vi "RVHR - Configure Language.vi"(7 "Directory Path":path, 8 "error in (no error)":errorcluster, 10 "Supervisory Config Cluster Out":T3={"UI Information"={"Header Image"=path "../Data/header.png", "Language"=enum."English", "First Run?"=FALSE, "Setup Camera?"=FALSE, "Device Type"=enum."RCA", "Encoder Type"=enum."Tacho", "Version"=enum."RailMeasurement_CAT", "port"=0, "greyscale"=FALSE, "camera index"=0}, "Test Cluster"={"Operator"="", "Description"="", "Line"="", "Start Position"=450000.0, "Run Length"=31.0, "Sensor A Position"=80000.0, "Rail Side"=FALSE, "Distance Direction"=FALSE, "Path"=path "", "Sensor B Position"=0.0, "Visible Chart Distance"=0.0, "Company"="", "Ref Profile"=""}, "RV-HR Settings Cluster"={"Sensor A Calibration"=0.0, "Integrator Time"=0.0, "Encoder Spacing"=0.0, "Encoder Threshold"=0.0, "Sampling Distance"=0, "Swap Direction?"=FALSE, "Min Walking Speed"=0.0, "Max Walking Speed"=0.0, "Distance Format"=0, "Sensor B Calibration"=0.0, "Tacho Pulses/Rev"=0.0, "Wheel Diameter"=0.0, "Max Short Roughness"=0.0, "Max Long Roughness"=0.0, "Measuring Interval"=0.0, "Measuring Length"=0.0, "Wavelengths"=[], "Device Resolution"=0, "Detect Change in Direction?"=FALSE, "Save Images?"=FALSE, "Image Frequency"=0, "Save Video?"=FALSE, "Image Offset"=0.0, "Start Position at 0m?"=FALSE, "Live Corrug Est.?"=FALSE, "Wavelength Corrug"=0, "Distance Corrug"=0, "Update Corrug"=0}} {"RV-HR Settings Cluster"."Image Frequency" items=["2", "3", "5"]; "RV-HR Settings Cluster"."Device Resolution" items=["0.1 µm", "1 µm", "10 µm"]; "RV-HR Settings Cluster"."Distance Format" items=["kilometres", "miles & chains", "metres", "stations", "miles"]; "RV-HR Settings Cluster"."Sampling Distance" items=["1mm", "2mm"]}, 11 "UI References":T13) -> (0 "error out":errorcluster, 1 "UI Information.Language":T1, 2 "Language Config Cluster Out":T2={"Home"="Home", "Test Setup"="Setup", "Run Test"="Test", "Configure"="Config", "Hardware Viewer"="Viewer", "Review Test"="Review", "Report"="Home", "Exit"="Exit", "Device Connected?"="Device Connected?", "Test in Progress?"="Test in Progress?", "Simulate?"="Simulate?", "Device Type 1"="Corrugation Analysis Trolley", "Device Type 2"="Bi-Corrugation Analysis Trolley", "Device Type 3"="Bi-Corrugation Analysis Trolley", "Device Type 4"="Bi-Corrugation Analysis Trolley", "Device Type 5"="Bi-Corrugation Analysis Trolley", "Device Type 6"="Bi-Corrugation Analysis Trolley", "Device Type 7"="Bi-Corrugation Analysis Trolley", "Software Version"="Version", "Support"="Software by RailMeasurement Limited - Cambridge - UK - support@railmeasurement.com", "Operator"="Operator:", "Test Description"="Description:", "Line"="Description:", "Test Folder Path"="Folder Path:", "Test Folder Path RCA"="Folder Path:", "Start Position"="Start Position:", "Sensor Position"="Sensor Position:", "Sensor A Position"="Sensor A Position:", "Sensor B Position"="Sensor B Position:", "Visible Chart Distance"="Sensor B Position:", "Rail Side"="Rail Side:", "Rail A Side"="Rail A Side:", "Distance Direction"="Distance Direction:", "Start"="Start:", "Distance Travelled"="Distance Travelled:", "Current Position"="Current Position:", "Stop Test"="Stop", "Pause Test"="Save", "Displacement"="Displacement", "Position"="Position", "Sensor Calibration"="Sensor Calibration:", "Sensor A Calibration"="Sensor A Calibration:", "Sensor B Calibration"="Sensor B Calibration:", "Encoder Spacing"="Encoder Spacing:", "Sampling Distance"="Sampling Distance:", "Tacho Pulses/Rev"="Sensor Calibration:", "Wheel Diameter"="Sensor A Calibration:", "Sampling Distances"=["1mm", "2mm"], "Distance Unit"="Distance in:", "Distance Units"=["Kilometres", "miles & chains", "metres", "stations", "miles"], "Swap Direction"="Swap Direction at Run End?", "Language"="Language", "Device Resolution"="Save", "Device Resolutions"=["Kilometres", "miles & chains", "metres", "stations", "miles"], "Detect Change in Direction"="Save", "Save Config"="Save", "Encoder Data"="Encoder Data", "Sensor Data"="Sensor Data", "Sensor A Data"="Sensor A Data", "Sensor B Data"="Sensor B Data", "Voltage"="Voltage", "Time (m:s)"="Time (m:s)", "Unit mm/s/V"="(mm/s)/V", "Unit mm"="mm", "Unit km"="km", "Unit m"="m", "Start Test Message"="m", "Stop Test Message"="km", "Exit Message"="mm", "File Exists Message"="mm", "File Path Invalid Message"="mm", "Combine Error"="mm", "Combine Success"="mm", "Roller Comp Error"="mm", "Test Folder Path (Live)"="mm", "Folder Error"="Sensor B Position:", "Enc Count"="Setup", "Run Start"="mm", "Run End"="mm", "Date"="mm", "Train"="Sensor B Position:", "Location"="Setup", "Notes"="mm", "Heading_1"="mm", "Heading_2"="mm", "Left Rail"="Sensor B Position:", "Right Rail"="Setup", "Left Exclusions"="mm", "Right Exclusions"="mm", "Settings"="mm", "Wavelength Ranges"="Sensor B Position:", "Y-Axis Limits"="Setup", "Exc Limits"="Sensor B Position:", "Other Settings"="Setup", "Distance/Page"="mm", "Distance/Pages"=["Kilometres", "miles & chains", "metres", "stations", "miles"], "Gridlines"="mm", "Report Tolerance"="mm", "Manual Cut"="Sensor B Position:", "Plot Colour"="Distance in:", "Plot Colours"=["Kilometres", "miles & chains", "metres", "stations", "miles"], "EN Standard"="mm", "RiL Standard"="mm", "Custom Standard"="mm", "Resolution"="Distance in:", "Resolutions"=["Kilometres", "miles & chains", "metres", "stations", "miles"], "Exceedence Header"="mm", "Distance (km)"="mm", "Left (%)"="mm", "Right (%)"="Distance in:", "Page"="Distance in:", "Align"="mm", "Main"="mm", "Comparison"="Distance in:", "Offset"="Distance in:", "From"="Distance in:", "To"="Distance in:", "Of"="Distance in:", "File"="mm", "Load New"="mm", "Load Comparison"="Distance in:", "Discard Comparison"="Distance in:", "Print Current Page"="Distance in:", "Print All Pages"="Distance in:", "Print Exceedence Report"="Distance in:", "Plot Main"="Distance in:", "No Comparison Data to Align"="Distance in:", "Run Load Error"="Distance in:", "Report Load Error"="Distance in:", "Cut"="Distance in:", "Remove"="Distance in:", "Config Settings Unsaved"="Distance in:", "Acquisition Paused"="Distance in:", "Please Select One Option Below"="Distance in:", "RCA is Now Stationary"="Distance in:", "Reporting Setting"="Distance in:", "Main Abbreviated"="Distance in:", "Comparison Abbreviated"="Distance in:", "Exceedence Abbreviated"="Distance in:", "Align Comparison"="Distance in:", "Rail Corrugation Analyser Reporting"="Distance in:", "Show Exc. % in Graph"="Distance in:", "Evaluate Sections <100m"="Distance in:", "Evaluate Sections <0.062mile"="Distance in:", "Section Too Short for Evaluation"="Distance in:", "Language Change Prompt"="Distance in:", "Show All"="Distance in:", "Sections_km"="Distance in:", "Sections_mi"="Distance in:", "Vision"="Distance in:", "Vision Report"="Distance in:", "Vision Display"="Distance in:", "Vision Displays"=["Kilometres", "miles & chains", "metres", "stations", "miles"], "Save Images"="Distance in:", "Image Frequency"="Distance in:", "Section"="Distance in:", "Brightness"="Distance in:", "Contrast"="Distance in:", "Shadow"="Distance in:", "Sharpened"="Distance in:", "Apply to all Images"="Distance in:", "Reset"="Distance in:", "Are you sure"="Distance in:", "Image Processing"="Distance in:", "Save Video"="Distance in:", "Image Offset"="Distance in:", "Camera Mode"="Distance in:", "Camera Modes"=["Kilometres", "miles & chains", "metres", "stations", "miles"], "Copy Page"="Distance in:", "Copy Graphs"="Distance in:", "Camera Mode Change Prompt"="Distance in:", "Camera_1 Missing"="Distance in:", "Camera_2 Missing"="Distance in:", "Cameras Missing"="Distance in:", "Camera Setup"="Distance in:", "Camera_1 Connection Error"="Distance in:", "Camera_2 Connection Error"="Distance in:", "Cameras Connection Error"="Distance in:", "No GPS"="Distance in:", "No Signal"="Distance in:", "Camera_1 Connected"="Distance in:", "Camera_1 Not Connected"="Distance in:", "Camera_2 Connected"="Distance in:", "Camera_2 Not Connected"="Distance in:", "Start Position at 0m?"="Distance in:", "Continue"="Distance in:", "New Test, Same Direction"="Distance in:", "New Test, Opposite Direction"="Distance in:", "Stop and Save"="Distance in:", "Live Corrug Estimate"="Distance in:", "Wavelength Corrug"="Distance in:", "Distance Corrug "="Distance in:", "Update Corrug"="Distance in:", "Company"="Distance in:", "Ref Profile "="Distance in:", "Company_Report"="Distance in:", "Ref Profile_Report"="Distance in:", "Heading_1_RVHR"="Distance in:", "Heading_2_RVHR"="Distance in:", "Remove Feature"="Distance in:", "Feature Type"="Sampling Distance:", "Feature Types"=["1mm", "2mm"], "AI Not Ready"="Sampling Distance:"}, 3 "Support":string)   [LabVIEW 2024]
uses:
  Controls/RVHR - UI Refs.ctl
  Controls/Supervisory Config Cluster.ctl
  Controls/UI Init Config Info.ctl
  Controls/Language.ctl
  Controls/Device_Type.ctl
  Controls/EncoderType.ctl
  Controls/Software Version.ctl
  Controls/Test Cluster.ctl
  Controls/Settings Cluster.ctl
  Controls/Sampling DIstance.ctl
  Controls/Distance Units.ctl
  Controls/Device_Resolution.ctl
  Controls/Language Vision Text Cluster.ctl
  <vilib>/addons/Tools/Unicode/UI Unicode Tools.lvlib
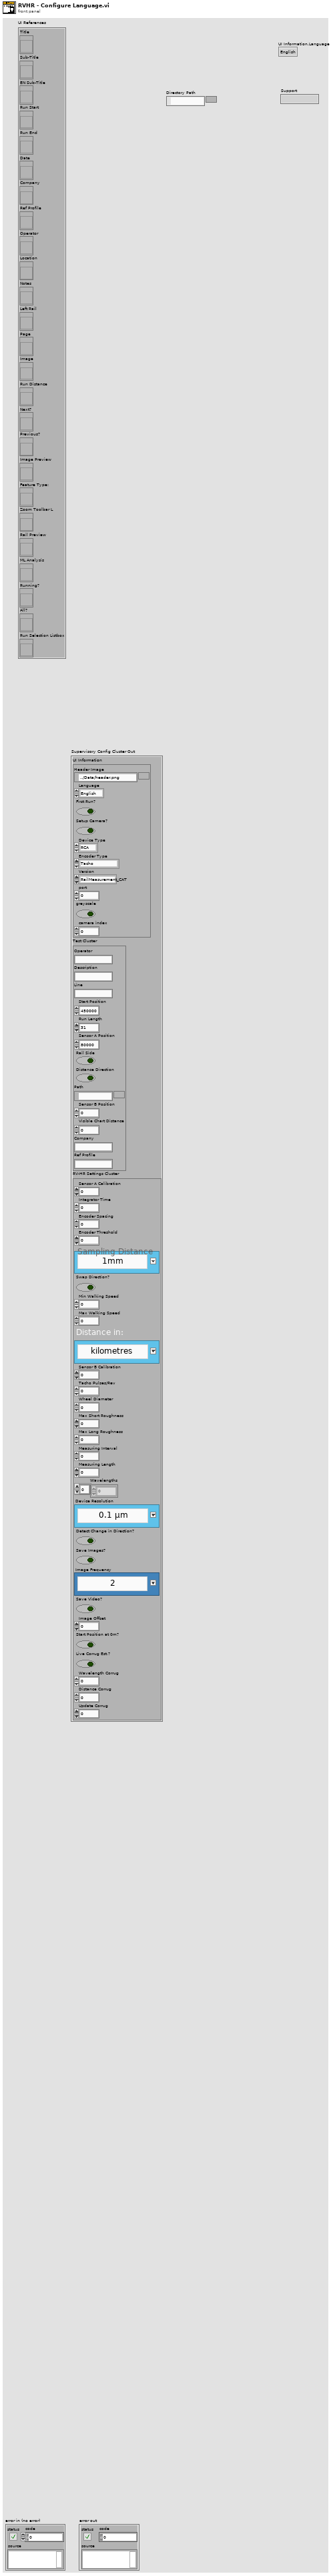
[diagram p1: front panel]
types:
  T1 = typedef "Language.ctl" = enum16{"English", "Chinese", "German"}
  T2 = typedef "Language Vision Text Cluster.ctl" = cluster{"Home":string, "Test Setup":string, "Run Test":string, "Configure":string, "Hardware Viewer":string, "Review Test":string, "Report":string, "Exit":string, "Device Connected?":string, "Test in Progress?":string, "Simulate?":string, "Device Type 1":string, "Device Type 2":string, "Device Type 3":string, "Device Type 4":string, "Device Type 5":string, "Device Type 6":string, "Device Type 7":string, "Software Version":string, "Support":string, "Operator":string, "Test Description":string, "Line":string, "Test Folder Path":string, "Test Folder Path RCA":string, "Start Position":string, "Sensor Position":string, "Sensor A Position":string, "Sensor B Position":string, "Visible Chart Distance":string, "Rail Side":string, "Rail A Side":string, "Distance Direction":string, "Start":string, "Distance Travelled":string, "Current Position":string, "Stop Test":string, "Pause Test":string, "Displacement":string, "Position":string, "Sensor Calibration":string, "Sensor A Calibration":string, "Sensor B Calibration":string, "Encoder Spacing":string, "Sampling Distance":string, "Tacho Pulses/Rev":string, "Wheel Diameter":string, "Sampling Distances":string[], "Distance Unit":string, "Distance Units":string[], "Swap Direction":string, "Language":string, "Device Resolution":string, "Device Resolutions":string[], "Detect Change in Direction":string, "Save Config":string, "Encoder Data":string, "Sensor Data":string, "Sensor A Data":string, "Sensor B Data":string, "Voltage":string, "Time (m:s)":string, "Unit mm/s/V":string, "Unit mm":string, "Unit km":string, "Unit m":string, "Start Test Message":string, "Stop Test Message":string, "Exit Message":string, "File Exists Message":string, "File Path Invalid Message":string, "Combine Error":string, "Combine Success":string, "Roller Comp Error":string, "Test Folder Path (Live)":string, "Folder Error":string, "Enc Count":string, "Run Start":string, "Run End":string, "Date":string, "Train":string, "Location":string, "Notes":string, "Heading_1":string, "Heading_2":string, "Left Rail":string, "Right Rail":string, "Left Exclusions":string, "Right Exclusions":string, "Settings":string, "Wavelength Ranges":string, "Y-Axis Limits":string, "Exc Limits":string, "Other Settings":string, "Distance/Page":string, "Distance/Pages":string[], "Gridlines":string, "Report Tolerance":string, "Manual Cut":string, "Plot Colour":string, "Plot Colours":string[], "EN Standard":string, "RiL Standard":string, "Custom Standard":string, "Resolution":string, "Resolutions":string[], "Exceedence Header":string, "Distance (km)":string, "Left (%)":string, "Right (%)":string, "Page":string, "Align":string, "Main":string, "Comparison":string, "Offset":string, "From":string, "To":string, "Of":string, "File":string, "Load New":string, "Load Comparison":string, "Discard Comparison":string, "Print Current Page":string, "Print All Pages":string, "Print Exceedence Report":string, "Plot Main":string, "No Comparison Data to Align":string, "Run Load Error":string, "Report Load Error":string, "Cut":string, "Remove":string, "Config Settings Unsaved":string, "Acquisition Paused":string, "Please Select One Option Below":string, "RCA is Now Stationary":string, "Reporting Setting":string, "Main Abbreviated":string, "Comparison Abbreviated":string, "Exceedence Abbreviated":string, "Align Comparison":string, "Rail Corrugation Analyser Reporting":string, "Show Exc. % in Graph":string, "Evaluate Sections <100m":string, "Evaluate Sections <0.062mile":string, "Section Too Short for Evaluation":string, "Language Change Prompt":string, "Show All":string, "Sections_km":string, "Sections_mi":string, "Vision":string, "Vision Report":string, "Vision Display":string, "Vision Displays":string[], "Save Images":string, "Image Frequency":string, "Section":string, "Brightness":string, "Contrast":string, "Shadow":string, "Sharpened":string, "Apply to all Images":string, "Reset":string, "Are you sure":string, "Image Processing":string, "Save Video":string, "Image Offset":string, "Camera Mode":string, "Camera Modes":string[], "Copy Page":string, "Copy Graphs":string, "Camera Mode Change Prompt":string, "Camera_1 Missing":string, "Camera_2 Missing":string, "Cameras Missing":string, "Camera Setup":string, "Camera_1 Connection Error":string, "Camera_2 Connection Error":string, "Cameras Connection Error":string, "No GPS":string, "No Signal":string, "Camera_1 Connected":string, "Camera_1 Not Connected":string, "Camera_2 Connected":string, "Camera_2 Not Connected":string, "Start Position at 0m?":string, "Continue":string, "New Test, Same Direction":string, "New Test, Opposite Direction":string, "Stop and Save":string, "Live Corrug Estimate":string, "Wavelength Corrug":string, "Distance Corrug ":string, "Update Corrug":string, "Company":string, "Ref Profile ":string, "Company_Report":string, "Ref Profile_Report":string, "Heading_1_RVHR":string, "Heading_2_RVHR":string, "Remove Feature":string, "Feature Type":string, "Feature Types":string[], "AI Not Ready":string}
  T3 = typedef "Supervisory Config Cluster.ctl" = cluster{"UI Information":T4, "Test Cluster":T8, "RV-HR Settings Cluster":T9}
  T4 = typedef "UI Init Config Info.ctl" = cluster{"Header Image":path, "Language":T1, "First Run?":bool, "Setup Camera?":bool, "Device Type":T5, "Encoder Type":T6, "Version":T7, "port":i32, "greyscale":bool, "camera index":i32}
  T5 = typedef "Device_Type.ctl" = enum16{"CAT", "Bi-CAT", "YRCA", "RCA", "RV-HR", "TV-HR"}
  T6 = typedef "EncoderType.ctl" = enum16{"Tacho", "Quadrature"}
  T7 = typedef "Software Version.ctl" = enum16{"RailMeasurement_CAT", "RailMeasurement_Master", "RailMeasurement_RCA", "RailMeasurement_CAT-V", "RailMeasurement_RCA-V", "RailMeasurement_RV-HR"}
  T8 = typedef "Test Cluster.ctl" = cluster{"Operator":string, "Description":string, "Line":string, "Start Position":dbl, "Run Length":dbl, "Sensor A Position":dbl, "Rail Side":bool, "Distance Direction":bool, "Path":path, "Sensor B Position":dbl, "Visible Chart Distance":dbl, "Company":string, "Ref Profile":string}
  T9 = typedef "Settings Cluster.ctl" = cluster{"Sensor A Calibration":dbl, "Integrator Time":dbl, "Encoder Spacing":dbl, "Encoder Threshold":dbl, "Sampling Distance":T10, "Swap Direction?":bool, "Min Walking Speed":dbl, "Max Walking Speed":dbl, "Distance Format":T11, "Sensor B Calibration":dbl, "Tacho Pulses/Rev":dbl, "Wheel Diameter":dbl, "Max Short Roughness":dbl, "Max Long Roughness":dbl, "Measuring Interval":dbl, "Measuring Length":dbl, "Wavelengths":dbl[], "Device Resolution":T12, "Detect Change in Direction?":bool, "Save Images?":bool, "Image Frequency":T10, "Save Video?":bool, "Image Offset":dbl, "Start Position at 0m?":bool, "Live Corrug Est.?":bool, "Wavelength Corrug":u8, "Distance Corrug":u8, "Update Corrug":u8}
  T10 = typedef "Sampling DIstance.ctl" = u16
  T11 = typedef "Distance Units.ctl" = u16
  T12 = typedef "Device_Resolution.ctl" = u16
  T13 = typedef "RVHR - UI Refs.ctl" = cluster{"Title":refnum<vi>, "Sub-Title":refnum<vi>, "EN Sub-Title":refnum<vi>, "Run Start":refnum<vi>, "Run End":refnum<vi>, "Date":refnum<vi>, "Company":refnum<vi>, "Ref Profile":refnum<vi>, "Operator":refnum<vi>, "Location":refnum<vi>, "Notes":refnum<vi>, "Left Rail":refnum<vi>, "Page":refnum<vi>, "Image":refnum<vi>, "Run Distance":refnum<vi>, "Next?":refnum<vi>, "Previous?":refnum<vi>, "Image Preview":refnum<vi>, "Feature Type:":refnum<vi>, "Zoom Toolbar L":refnum<vi>, "Rail Preview":refnum<vi>, "ML Analysis":refnum<vi>, "Running?":refnum<vi>, "All?":refnum<vi>, "Run Selection Listbox":refnum<vi>}
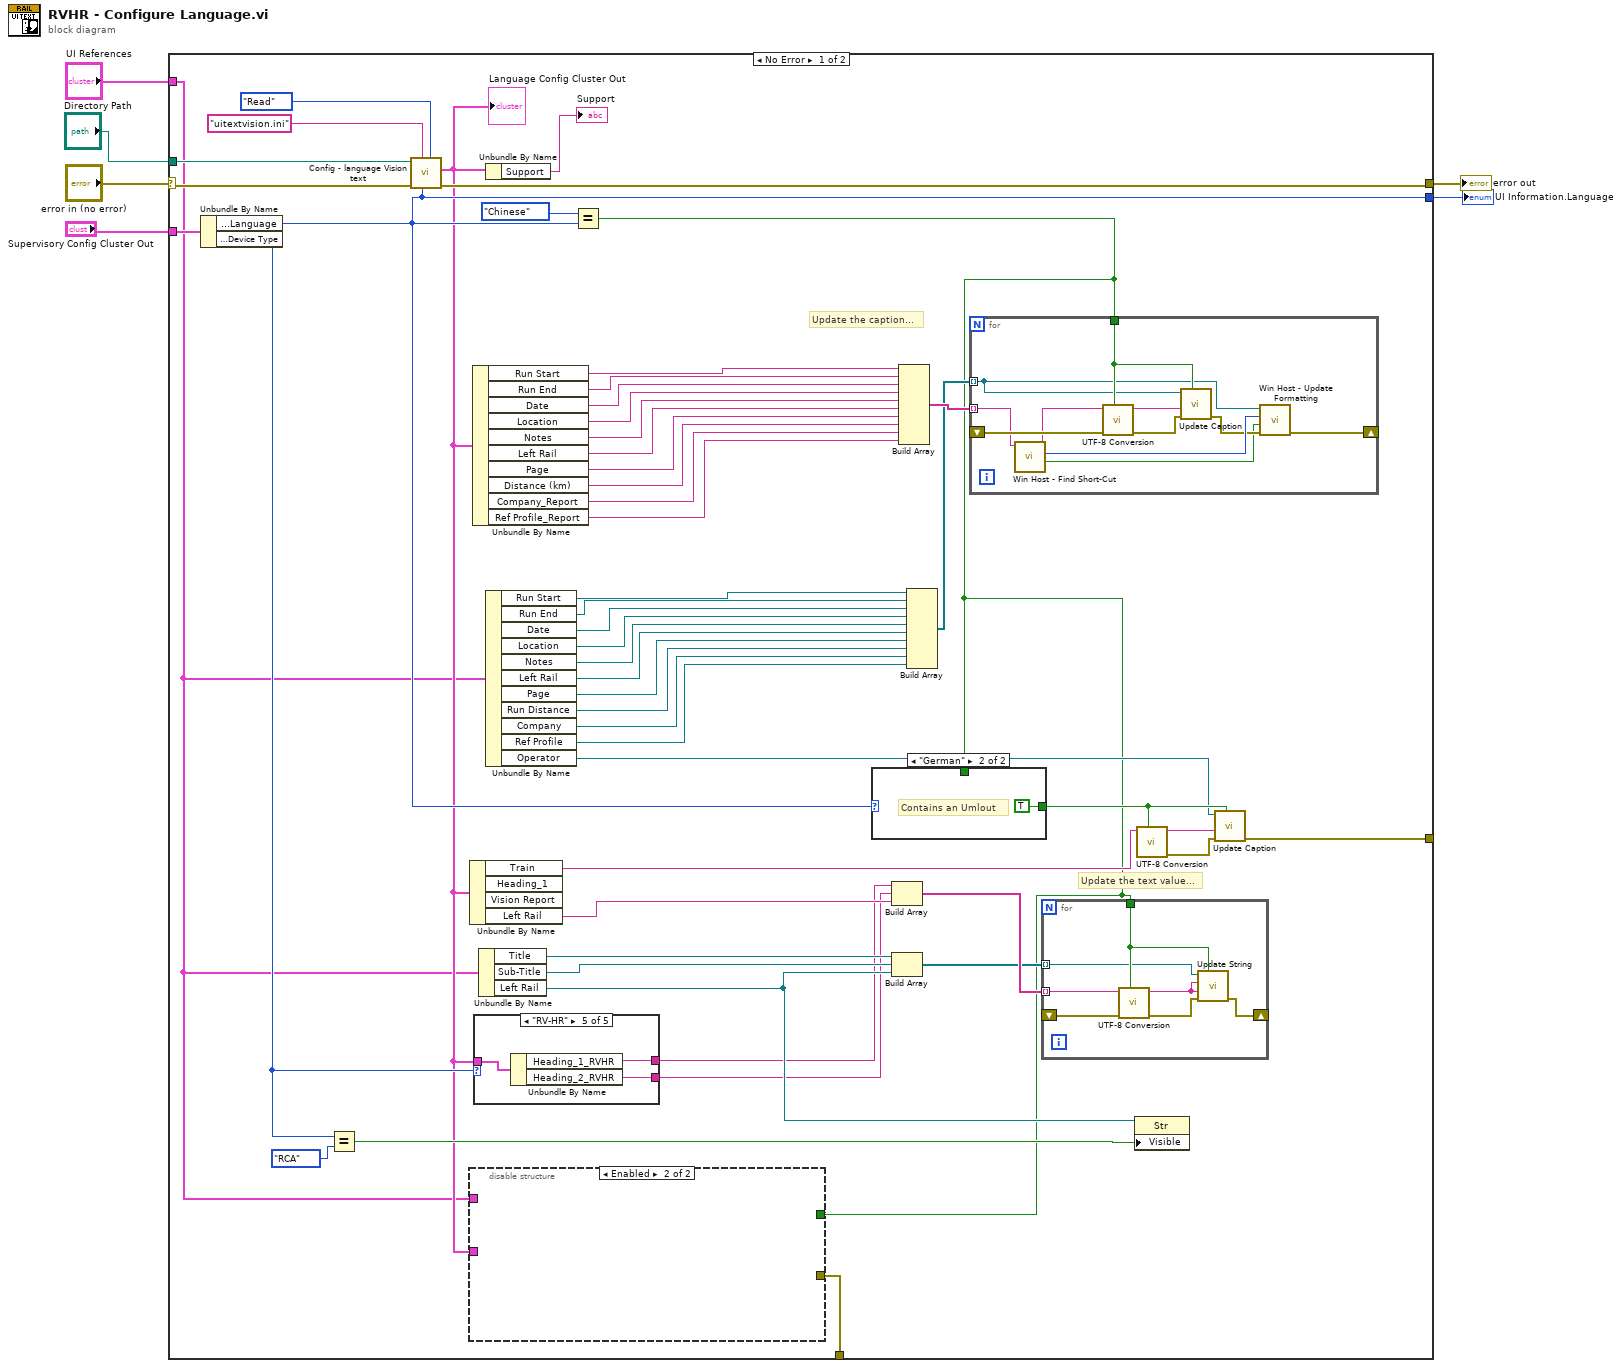
[diagram p0: block diagram]
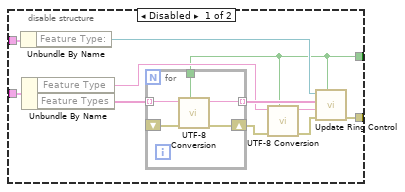
[diagram p2: hidden frame]
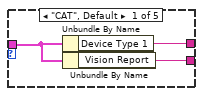
[diagram p3: hidden frame]
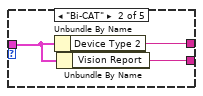
[diagram p4: hidden frame]
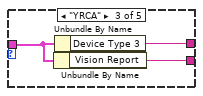
[diagram p5: hidden frame]
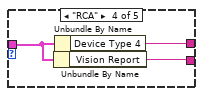
[diagram p6: hidden frame]
diagram:
  n1 = case shown="No Error" "error in (no error)" {
    selector: "error in (no error)" -> [w58 w110]
    tunnel: [w57 w110] -> w5
    tunnel: "UI References" -> [w10 _]
    tunnel: "Supervisory Config Cluster Out" -> [w51 _]
    tunnel: "Directory Path" -> [w52 _]
    tunnel: [w50 _] -> w1
    tunnel: [w8 _] -> _
    tunnel: [w7 _] -> _
    frame No Error {
      # "Update the caption..."
      # "Update the text value..."
      n2 = Unbundle By Name(w51) -> ("UI Information.Language"=w50:T1, "UI Information.Device Type"=w18:T5)
      n3 = Equal?(x=w18, y=Device_Type."RCA") -> (x = y?=w19:bool)
      n4 = call "Config - language Vision text.vi"(".ini Controller"=enum16{"Read", "Write"}."Read", "Language"=w50, ".ini filename"="uitextvision.ini", "error in (no error)"=w58, "Directory Path"=w52) -> ("error out"=w57:errorcluster, "Language Config Cluster Out"=w11:T2)  [unwired: 4 in, 1 out]
      "Language Config Cluster Out" <- w11
      n5 = Unbundle By Name(w11) -> ("Train"=w24:string, "Left Rail"=w29:string)  [unwired: 2 out]
      n6 = Unbundle By Name(w11) -> ("Run Start"=w40:string, "Run End"=w39:string, "Date"=w38:string, "Location"=w37:string, "Notes"=w36:string, "Left Rail"=w35:string, "Page"=w34:string, "Distance (km)"=w23:string, "Company_Report"=w14:string, "Ref Profile_Report"=w13:string)
      n7 = case shown="\"RV-HR\"" w18 {
        tunnel: w11 -> [w76 w79 w82 w85 w89]
        tunnel: [w77 w80 w83 w86 w88] -> w17
        tunnel: [w75 w78 w81 w84 w87] -> w12
        frame "CAT", Default {
          n8 = Unbundle By Name(w76) -> ("Device Type 1"=w77:string)
          n9 = Unbundle By Name(w76) -> ("Vision Report"=w75:string)
        }
        frame "Bi-CAT" {
          n10 = Unbundle By Name(w79) -> ("Device Type 2"=w80:string)
          n11 = Unbundle By Name(w79) -> ("Vision Report"=w78:string)
        }
        frame "YRCA" {
          n12 = Unbundle By Name(w82) -> ("Vision Report"=w81:string)
          n13 = Unbundle By Name(w82) -> ("Device Type 3"=w83:string)
        }
        frame "RCA" {
          n14 = Unbundle By Name(w85) -> ("Vision Report"=w84:string)
          n15 = Unbundle By Name(w85) -> ("Device Type 4"=w86:string)
        }
        frame "RV-HR" {
          n16 = Unbundle By Name(w89) -> ("Heading_1_RVHR"=w88:string, "Heading_2_RVHR"=w87:string)
        }
      }
      n17 = Unbundle By Name(w10) -> ("Title"=w30:refnum<vi>, "Sub-Title"=w31:refnum<vi>, "Left Rail"=w21:refnum<vi>)
      n18 = Unbundle By Name(w11) -> ("Support"=→"Support":string)
      n19 = Unbundle By Name(w10) -> ("Run Start"=w47:refnum<vi>, "Run End"=w46:refnum<vi>, "Date"=w45:refnum<vi>, "Location"=w44:refnum<vi>, "Notes"=w43:refnum<vi>, "Left Rail"=w42:refnum<vi>, "Page"=w41:refnum<vi>, "Run Distance"=w22:refnum<vi>, "Company"=w16:refnum<vi>, "Ref Profile"=w15:refnum<vi>, "Operator"=w25:refnum<vi>)
      n20 = Equal?(x=Language."Chinese" ("UI Information.Language"), y=w50) -> (x = y?=w9:bool)
      n21 = disable-structure shown="Enabled" {
        disable-tunnel: w11 -> [w65 _]
        disable-tunnel: w10 -> [w62 _]
        disable-tunnel: w9 -> [w59 _]
        disable-tunnel: [w60 _] -> w8
        frame Disabled {
          n22 = Unbundle By Name(w62) -> ("Feature Type:"=w61:refnum<vi>)
          n23 = Unbundle By Name(w65) -> ("Feature Type"=w63:string, "Feature Types"=w64:string[])
          n24 = for {
            shift-right: [w73] -> w67
            shift-left: _ -> [w74]
            tunnel: [w72] -> w69 mode=indexing
            tunnel: w64 -> [w71] mode=indexing
            tunnel: w59 -> [w70]
            n25 = call "UTF-8 Conversion.vi"("Unicode?"=w70, "error in"=w74, "Config String"=w71) -> ("error out"=w73:errorcluster, "Unicode/ANSI string"=w72:string)  [unwired: 7 in]
          }
          n26 = call "UTF-8 Conversion.vi"("Unicode?"=w59, "error in"=w67, "Config String"=w63) -> ("error out"=w66:errorcluster, "Unicode/ANSI string"=w68:string)  [unwired: 7 in]
          n27 = call <vilib>:"Update Ring Control.vi"("Interpret as Unicode (T)"=w59, "error in (no error)"=w66, "Caption"=w68, "Strings"=w69, "Ring Control Ref"=w61) -> ("error out"=w60:errorcluster)  [unwired: 4 in]
        }
        frame Enabled {
        }
      }
      n28 = case shown="\"German\"" w50 {
        tunnel: w9 -> [w101 _]
        tunnel: [w101 TRUE] -> w26
        frame "English", Default {
        }
        frame "German" {
          # "Contains an Umlout"
        }
      }
      n29 = Build Array(w17, w12, w29) -> (w33:string[])
      n30 = Build Array(w30, w31, w21) -> (w32:refnum<vi>[])
      n31 = Build Array(w40, w39, w38, w37, w36, w35, w34, w23, w14, w13) -> (w49:string[])
      n32 = Build Array(w47, w46, w45, w44, w43, w42, w41, w22, w16, w15) -> (w48:refnum<vi>[])
      n33 = for {
        tunnel: w49 -> [w96] mode=indexing
        tunnel: w9 -> [w99]
        tunnel: w48 -> [w93] mode=indexing
        shift-right: [w91] -> _
        shift-left: _ -> [w97]
        n34 = call "Win Host - Find Short-Cut.vi"("Language in"=w96) -> ("Short-Cut?"=w90:bool, "S/CUT Index"=w94:i32, "Language out"=w95:string)  [unwired: 8 in]
        n35 = call "UTF-8 Conversion.vi"("Unicode?"=w99, "error in"=w97, "Config String"=w95) -> ("error out"=w98:errorcluster, "Unicode/ANSI string"=w100:string)  [unwired: 7 in]
        n36 = call <vilib>:"Update Caption.vi"("Interpret as Unicode (T)"=w99, "error in (no error)"=w98, "Caption"=w100, "Control Reference"=w93) -> ("error out"=w92:errorcluster)  [unwired: 4 in, 1 out]
        n37 = call "Win Host - Update Formatting.vi"("error in (no error)"=w92, "Short-Cut?"=w90, "Index"=w94, "Control in"=w93) -> ("error out"=w91:errorcluster)  [unwired: 7 in]
      }
      n38 = for {
        tunnel: w33 -> [w104] mode=indexing
        tunnel: w9 -> [w106]
        tunnel: w32 -> [w105] mode=indexing
        shift-right: [w107] -> _
        shift-left: _ -> [w109]
        n39 = call "UTF-8 Conversion.vi"("Unicode?"=w106, "error in"=w109, "Config String"=w104) -> ("error out"=w108:errorcluster, "Unicode/ANSI string"=w103:string)  [unwired: 7 in]
        n40 = call <vilib>:"Update String.vi"("Interpret as Unicode (T)"=w106, "error in (no error)"=w108, "Caption"=w103, "String Value"=w103, "String Control Reference"=w105) -> ("error out"=w107:errorcluster)  [unwired: 3 in, 1 out]
      }
      n41 = property class="Str"(reference=w21, "Visible"=w19) -> ()  [unwired: 1 in, 2 out]
      n42 = call "UTF-8 Conversion.vi"("Unicode?"=w26, "Config String"=w24) -> ("error out"=w28:errorcluster, "Unicode/ANSI string"=w27:string)  [unwired: 8 in]
      n43 = call <vilib>:"Update Caption.vi"("Interpret as Unicode (T)"=w26, "error in (no error)"=w28, "Caption"=w27, "Control Reference"=w25) -> ("error out"=w7:errorcluster)  [unwired: 4 in, 1 out]
    }
    frame Error {
    }
  }
  "error out" <- w5
  "UI Information.Language" <- w1
